vi "E364XA Console 2.vi"() -> ()   [LabVIEW 2010]
panel:
  in  "Volt":dbl
  out "Sel Chn Dly":bool
  in  "Sel Chn":bool
  out "Current":dbl
  out "Voltage":dbl
  in  "Set":bool
  in  "Stop":bool
  out "Current":string
  out "Voltage":string
  in  "VISA session":refnum<visa-resource-name>="COM9"
  in  "OFF SW":bool
  out "OFF":bool
  in  "ON SW":bool
  out "ON":bool
  out "error out":errorcluster
  in  "error in (no error)":errorcluster
  # "Agilent Console 2"
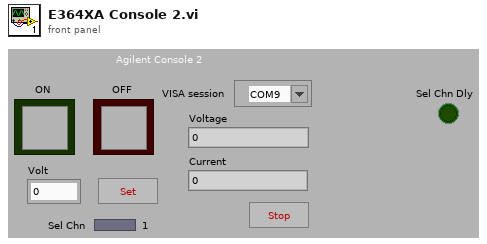
[diagram p1: front panel]
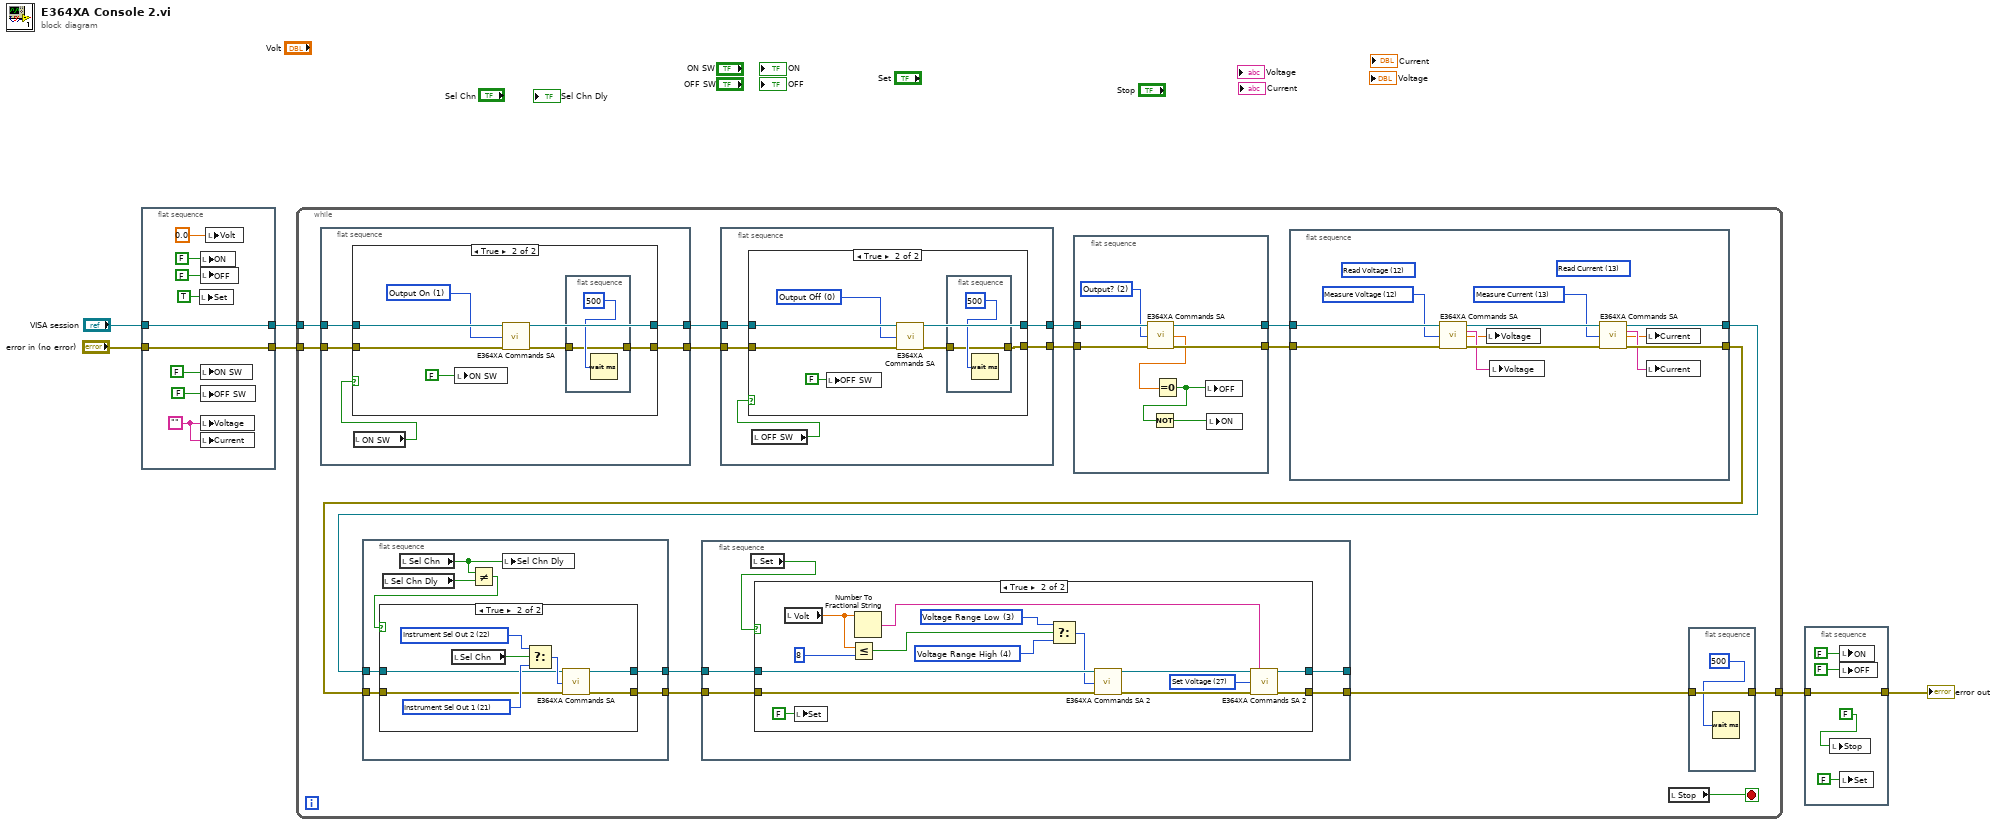
[diagram p0: block diagram]
diagram:
  n1 = flat-sequence {
    tunnel: [w15] -> w3
    tunnel: "error in (no error)" -> [w15]
    tunnel: [w14] -> w1
    tunnel: "VISA session" -> [w14]
    frame #0 {
      w9 = ""
      n2 = local write "Set"(TRUE ("Set")) -> ()
      n3 = local write "ON"(FALSE) -> ()
      n4 = local write "OFF"(FALSE) -> ()
      n5 = local write "ON SW"(FALSE) -> ()
      n6 = local write "OFF SW"(FALSE) -> ()
      n7 = local write "Voltage"(w9) -> ()
      n8 = local write "Current"(w9) -> ()
      n9 = local write "Volt"(0.0) -> ()
    }
  }
  n10 = while {
    tunnel: w1 -> [w26]
    tunnel: w3 -> [w25]
    tunnel: [w27] -> w6
    stop <- w28 stop-if-true
    n11 = flat-sequence {
      tunnel: w26 -> [w112]
      tunnel: w25 -> [w111]
      tunnel: [w110] -> w30
      tunnel: [w109] -> w29
      frame #0 {
        n12 = local read "ON SW"() -> (w108:bool)
        n13 = case shown="True" w108 {
          tunnel: w112 -> [w114 w119]
          tunnel: w111 -> [w113 w120]
          tunnel: [w114 w117] -> w110
          tunnel: [w113 w121] -> w109
          frame False {
          }
          frame True {
            w118 = u16 1 items=["Output Off", "Output On", "Output?", "Voltage Range Low", "Voltage Range High", "Voltage Range?", "Apply 12V, 1.5A", "Apply?", "Voltage 12V", "Voltage?", "Current 1.5A", "Current?", "Measure Voltage", "Measure Current", "Set RS232", "Set Remote Mode", "Set Local Mode", "System Error?", "*IDN?", "*RST", "Instrument Sel?", "Instrument Sel Out 1", "Instrument Sel Out 2", "Display Mode VI", "Display Mode VV", "Display Mode II", "Apply 0V, 0A"] ("Command")
            n14 = local write "ON SW"(FALSE) -> ()
            n15 = call "E364XA Commands SA.vi"("VISA session"=w119, "Command"=w118, "error in (no error)"=w120) -> ("VISA session out"=w117:refnum<visa-resource-name>, "error out"=w116:errorcluster)  [unwired: 7 in, 4 out]
            n16 = flat-sequence {
              tunnel: [w122] -> w121
              tunnel: w116 -> [w122]
              frame #0 {
                n17 = Wait (ms)(milliseconds to wait=500) -> ()  [unwired: 1 out]
              }
            }
          }
        }
      }
    }
    n18 = flat-sequence {
      tunnel: w20 -> [w59]
      tunnel: w19 -> [w58]
      tunnel: [w54] -> w18
      tunnel: [w53] -> w17
      frame #0 {
        n19 = local read "Sel Chn Dly"() -> (w57:bool)
        n20 = local read "Sel Chn"() -> (w56:bool)
        n21 = Not Equal?(x=w56, y=w57) -> (x != y?=w55:bool)
        n22 = case shown="True" w55 {
          tunnel: w59 -> [w60 w65]
          tunnel: w58 -> [w61 w64]
          tunnel: [w61 w63] -> w54
          tunnel: [w60 w62] -> w53
          frame False {
          }
          frame True {
            w67 = u16 21 items=["Output Off", "Output On", "Output?", "Voltage Range Low", "Voltage Range High", "Voltage Range?", "Apply 12V, 1.5A", "Apply?", "Voltage 12V", "Voltage?", "Current 1.5A", "Current?", "Measure Voltage", "Measure Current", "Set RS232", "Set Remote Mode", "Set Local Mode", "System Error?", "*IDN?", "*RST", "Instrument Sel?", "Instrument Sel Out 1", "Instrument Sel Out 2", "Display Mode VI", "Display Mode VV", "Display Mode II", "Apply 0V, 0A"] ("Command")
            w68 = u16 22 items=["Output Off", "Output On", "Output?", "Voltage Range Low", "Voltage Range High", "Voltage Range?", "Apply 12V, 1.5A", "Apply?", "Voltage 12V", "Voltage?", "Current 1.5A", "Current?", "Measure Voltage", "Measure Current", "Set RS232", "Set Remote Mode", "Set Local Mode", "System Error?", "*IDN?", "*RST", "Instrument Sel?", "Instrument Sel Out 1", "Instrument Sel Out 2", "Display Mode VI", "Display Mode VV", "Display Mode II", "Apply 0V, 0A"] ("Command")
            n23 = local read "Sel Chn"() -> (w66:bool)
            n24 = Select(t=w68, s=w66, f=w67) -> (s? t:f=w69:u16)
            n25 = call "E364XA Commands SA.vi"("VISA session"=w64, "Command"=w69, "error in (no error)"=w65) -> ("VISA session out"=w63:refnum<visa-resource-name>, "error out"=w62:errorcluster)  [unwired: 7 in, 4 out]
          }
        }
        n26 = local write "Sel Chn Dly"(w56) -> ()
      }
    }
    n27 = flat-sequence {
      tunnel: w18 -> [w35]
      tunnel: w17 -> [w34]
      tunnel: [w32] -> _
      tunnel: [w31] -> w16
      frame #0 {
        n28 = local read "Set"() -> (w33:bool)
        n29 = case shown="True" w33 {
          tunnel: w35 -> [w37 w45]
          tunnel: w34 -> [w36 w46]
          tunnel: [w37 w50] -> w32
          tunnel: [w36 w49] -> w31
          frame False {
          }
          frame True {
            w48 = u16 3 items=["Output Off", "Output On", "Output?", "Voltage Range Low", "Voltage Range High", "Voltage Range?", "Apply 12V, 1.5A", "Apply?", "Voltage 12V", "Voltage?", "Current 1.5A", "Current?", "Measure Voltage", "Measure Current", "Set RS232", "Set Remote Mode", "Set Local Mode", "System Error?", "*IDN?", "*RST", "Instrument Sel?", "Instrument Sel Out 1", "Instrument Sel Out 2", "Display Mode VI", "Display Mode VV", "Display Mode II", "Apply 0V, 0A", "Set Voltage"] ("Command")
            w47 = u16 4 items=["Output Off", "Output On", "Output?", "Voltage Range Low", "Voltage Range High", "Voltage Range?", "Apply 12V, 1.5A", "Apply?", "Voltage 12V", "Voltage?", "Current 1.5A", "Current?", "Measure Voltage", "Measure Current", "Set RS232", "Set Remote Mode", "Set Local Mode", "System Error?", "*IDN?", "*RST", "Instrument Sel?", "Instrument Sel Out 1", "Instrument Sel Out 2", "Display Mode VI", "Display Mode VV", "Display Mode II", "Apply 0V, 0A", "Set Voltage"] ("Command")
            w52 = u16 27 items=["Output Off", "Output On", "Output?", "Voltage Range Low", "Voltage Range High", "Voltage Range?", "Apply 12V, 1.5A", "Apply?", "Voltage 12V", "Voltage?", "Current 1.5A", "Current?", "Measure Voltage", "Measure Current", "Set RS232", "Set Remote Mode", "Set Local Mode", "System Error?", "*IDN?", "*RST", "Instrument Sel?", "Instrument Sel Out 1", "Instrument Sel Out 2", "Display Mode VI", "Display Mode VV", "Display Mode II", "Apply 0V, 0A", "Set Voltage"] ("Command")
            n30 = local read "Volt"() -> (w41:dbl)
            n31 = local write "Set"(FALSE ("Set")) -> ()
            n32 = Less Or Equal?(x=w41, y=8) -> (x <= y?=w39:bool)
            n33 = Number To Fractional String(number=w41) -> (F-format string=w38:string)  [unwired: 3 in]
            n34 = Select(t=w48, s=w39, f=w47) -> (s? t:f=w43:u16)
            n35 = call "E364XA Commands SA 2.vi"("VISA session"=w45, "Command"=w43, "error in (no error)"=w46) -> ("VISA session out"=w42:refnum<visa-resource-name>, "error out"=w44:errorcluster)  [unwired: 7 in, 4 out]
            n36 = call "E364XA Commands SA 2.vi"("VISA session"=w42, "Voltage"=w38, "Command"=w52, "error in (no error)"=w44) -> ("VISA session out"=w50:refnum<visa-resource-name>, "error out"=w49:errorcluster)  [unwired: 6 in, 4 out]
          }
        }
      }
    }
    n37 = flat-sequence {
      tunnel: w30 -> [w96]
      tunnel: w29 -> [w95]
      tunnel: [w94] -> w23
      tunnel: [w93] -> w24
      frame #0 {
        n38 = local read "OFF SW"() -> (w92:bool)
        n39 = case shown="True" w92 {
          tunnel: w96 -> [w98 w105]
          tunnel: w95 -> [w97 w104]
          tunnel: [w98 w103] -> w94
          tunnel: [w97 w101] -> w93
          frame False {
          }
          frame True {
            w100 = u16 0 items=["Output Off", "Output On", "Output?", "Voltage Range Low", "Voltage Range High", "Voltage Range?", "Apply 12V, 1.5A", "Apply?", "Voltage 12V", "Voltage?", "Current 1.5A", "Current?", "Measure Voltage", "Measure Current", "Set RS232", "Set Remote Mode", "Set Local Mode", "System Error?", "*IDN?", "*RST", "Instrument Sel?", "Instrument Sel Out 1", "Instrument Sel Out 2", "Display Mode VI", "Display Mode VV", "Display Mode II", "Apply 0V, 0A"] ("Command")
            n40 = local write "OFF SW"(FALSE) -> ()
            n41 = call "E364XA Commands SA.vi"("VISA session"=w105, "Command"=w100, "error in (no error)"=w104) -> ("VISA session out"=w103:refnum<visa-resource-name>, "error out"=w102:errorcluster)  [unwired: 7 in, 4 out]
            n42 = flat-sequence {
              tunnel: [w106] -> w101
              tunnel: w102 -> [w106]
              frame #0 {
                n43 = Wait (ms)(milliseconds to wait=500) -> ()  [unwired: 1 out]
              }
            }
          }
        }
      }
    }
    n44 = flat-sequence {
      tunnel: w23 -> [w77]
      tunnel: w24 -> [w76]
      tunnel: [w75] -> w22
      tunnel: [w74] -> w21
      frame #0 {
        w73 = u16 2 items=["Output Off", "Output On", "Output?", "Voltage Range Low", "Voltage Range High", "Voltage Range?", "Apply 12V, 1.5A", "Apply?", "Voltage 12V", "Voltage?", "Current 1.5A", "Current?", "Measure Voltage", "Measure Current", "Set RS232", "Set Remote Mode", "Set Local Mode", "System Error?", "*IDN?", "*RST", "Instrument Sel?", "Instrument Sel Out 1", "Instrument Sel Out 2", "Display Mode VI", "Display Mode VV", "Display Mode II", "Apply 0V, 0A"] ("Command")
        n45 = call "E364XA Commands SA.vi"("VISA session"=w77, "Command"=w73, "error in (no error)"=w76) -> ("VISA session out"=w75:refnum<visa-resource-name>, "Num Resp"=w72:dbl, "error out"=w74:errorcluster)  [unwired: 7 in, 3 out]
        n46 = Equal To 0?(x=w72) -> (x = 0?=w71:bool)
        n47 = Not(x=w71) -> (.not. x?=w70:bool)
        n48 = local write "OFF"(w71) -> ()
        n49 = local write "ON"(w70) -> ()
      }
    }
    n50 = flat-sequence {
      tunnel: [w91] -> w20
      tunnel: w22 -> [w90]
      tunnel: w21 -> [w89]
      tunnel: [w80] -> w19
      frame #0 {
        w83 = u16 13 items=["Output Off", "Output On", "Output?", "Voltage Range Low", "Voltage Range High", "Voltage Range?", "Apply 12V, 1.5A", "Apply?", "Voltage 12V", "Voltage?", "Current 1.5A", "Current?", "Measure Voltage", "Measure Current", "Set RS232", "Set Remote Mode", "Set Local Mode", "System Error?", "*IDN?", "*RST", "Instrument Sel?", "Instrument Sel Out 1", "Instrument Sel Out 2", "Display Mode VI", "Display Mode VV", "Display Mode II", "Apply 0V, 0A"] ("Command")
        w84 = u16 12 items=["Output Off", "Output On", "Output?", "Voltage Range Low", "Voltage Range High", "Voltage Range?", "Apply 12V, 1.5A", "Apply?", "Voltage 12V", "Voltage?", "Current 1.5A", "Current?", "Measure Voltage", "Measure Current", "Set RS232", "Set Remote Mode", "Set Local Mode", "System Error?", "*IDN?", "*RST", "Instrument Sel?", "Instrument Sel Out 1", "Instrument Sel Out 2", "Display Mode VI", "Display Mode VV", "Display Mode II", "Apply 0V, 0A"] ("Command")
        (unwired) u16 13 items=["Standby Mode", "Operating Mode", "Set Voltage", "Set Current", "Set Time", "Set OVP", "Disable OCP", "Enable OCP", "Store", "Recall", "Enable ATS", "Read All Data", "Read Voltage", "Read Current", "Read OCP", "Read OVP", "Read Time", "Read Status"] ("Command")
        (unwired) u16 12 items=["Standby Mode", "Operating Mode", "Set Voltage", "Set Current", "Set Time", "Set OVP", "Disable OCP", "Enable OCP", "Store", "Recall", "Enable ATS", "Read All Data", "Read Voltage", "Read Current", "Read OCP", "Read OVP", "Read Time", "Read Status"] ("Command")
        n51 = call "E364XA Commands SA.vi"("VISA session"=w90, "Command"=w84, "error in (no error)"=w89) -> ("VISA session out"=w88:refnum<visa-resource-name>, "Response"=w86:string, "Num Resp"=w82:dbl, "error out"=w87:errorcluster)  [unwired: 7 in, 2 out]
        n52 = local write "Voltage"(w82) -> ()
        n53 = local write "Voltage"(w86) -> ()
        n54 = call "E364XA Commands SA.vi"("VISA session"=w88, "Command"=w83, "error in (no error)"=w87) -> ("VISA session out"=w80:refnum<visa-resource-name>, "Response"=w85:string, "Num Resp"=w81:dbl, "error out"=w91:errorcluster)  [unwired: 7 in, 2 out]
        n55 = local write "Current"(w81) -> ()
        n56 = local write "Current"(w85) -> ()
      }
    }
    n57 = local read "Stop"() -> (w28:bool)
    n58 = flat-sequence {
      tunnel: w16 -> [w79]
      tunnel: [w79] -> w27
      frame #0 {
        n59 = Wait (ms)(milliseconds to wait=500) -> ()  [unwired: 1 out]
      }
    }
  }
  n60 = flat-sequence {
    tunnel: [w128] -> w5
    tunnel: w6 -> [w128]
    frame #0 {
      n61 = local write "Stop"(FALSE) -> ()
      n62 = local write "ON"(FALSE) -> ()
      n63 = local write "OFF"(FALSE) -> ()
      n64 = local write "Set"(FALSE ("Set")) -> ()
    }
  }
  "error out" <- w5
